vi "cal_cmd_to_string_position.vi"(0 "Last Function Ref In":refnum<vi>, 1 "Disable String":string="OFF", 2 "Enum":T1, 5 "Main Node BD Position":cluster{"Left":i32, "Top":i32}, 7 "1st sub node x position":i32, 9 "Last sub node y position/Offset":i32, 11 "error in (no error)":errorcluster) -> (4 "Last Function Ref Out":refnum<vi>, 6 "Main Node Position/Enable Constant Position":cluster{"Left":u32, "Top":i32}, 8 "Disable Constant Position":cluster{u32, i32}, 10 "1st sub node x position":i32, 15 "error out":errorcluster)   [LabVIEW 2018]
uses:
  TypeDefinitions/main_position_types.ctl
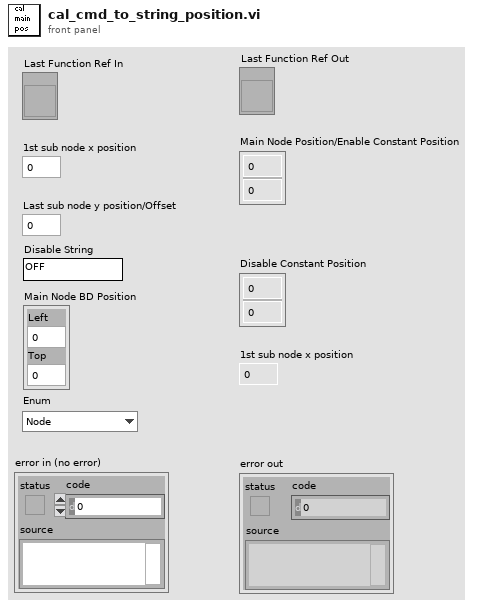
[diagram p1: front panel]
types:
  T1 = typedef "main_position_types.ctl" = enum16{"Node", "FormatNodeForMultipleControls", "BoolConstant", "FormatConstant", "1stSubNodeX"}
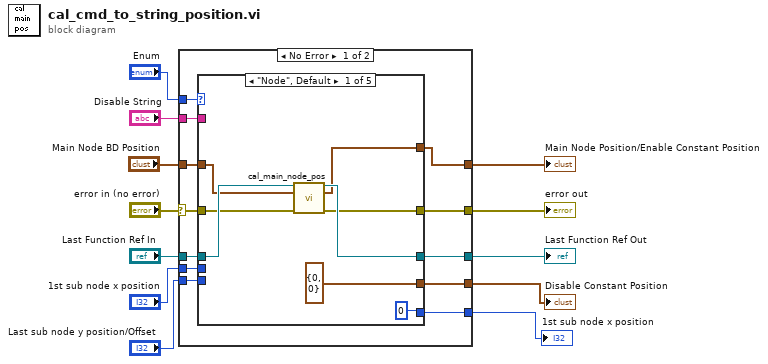
[diagram p0: block diagram]
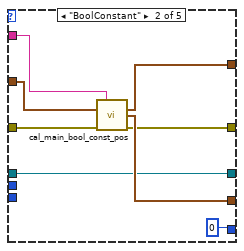
[diagram p2: hidden frame]
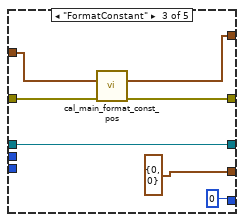
[diagram p3: hidden frame]
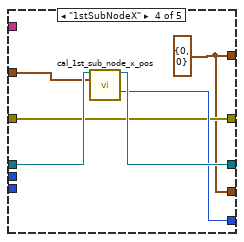
[diagram p4: hidden frame]
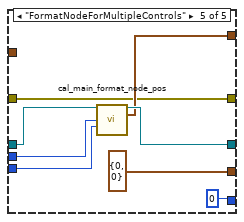
[diagram p5: hidden frame]
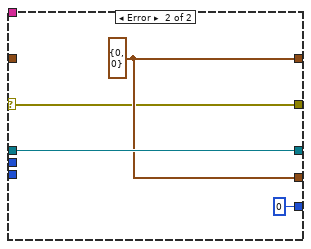
[diagram p6: hidden frame]
diagram:
  n1 = case shown="No Error" "error in (no error)" {
    selector: "error in (no error)" -> [w23 w63]
    tunnel: "Enum" -> [w24 _]
    tunnel: "Last Function Ref In" -> [w22 w65]
    tunnel: [w21 w65] -> w9
    tunnel: [w20 w64] -> w8
    tunnel: "1st sub node x position" -> [w19 _]
    tunnel: "Last sub node y position/Offset" -> [w18 _]
    tunnel: [w17 w63] -> w5
    tunnel: "Main Node BD Position" -> [w14 _]
    tunnel: "Disable String" -> [w16 _]
    tunnel: [w15 w64] -> w2
    tunnel: [w13 0 ("1st sub node x position")] -> w1
    frame No Error {
      n2 = case shown="\"Node\", Default" w24 {
        tunnel: w23 -> [w29 w36 w46 w49 w56]
        tunnel: w22 -> [w32 w34 w47 w53 w61]
        tunnel: [w31 w34 w47 w52 w60] -> w21
        tunnel: [w27 w38 w43 w48 w59] -> w20
        tunnel: w19 -> [_ _ _ _ w58]
        tunnel: w18 -> [_ _ _ _ w57]
        tunnel: [w28 w35 w45 w49 w56] -> w17
        tunnel: w14 -> [w30 w39 w44 w50 _]
        tunnel: w16 -> [_ w40 _ _ _]
        tunnel: [cluster{"Left":i32, "Top":i32} {"Left"=0, "Top"=0} ("Constant Position") w37 cluster{"Left":u32, "Top":i32} {"Left"=0, "Top"=0} ("Main Node Position") w48 cluster{"Left":i32, "Top":i32} {"Left"=0, "Top"=0} ("Constant Position")] -> w15
        tunnel: [0 ("1st sub node x position") 0 ("1st sub node x position") 0 ("1st sub node x position") w51 0 ("1st sub node x position")] -> w13
        frame "Node", Default {
          n3 = call "cal_main_node_pos.vi"("Last Function Ref"=w32, "Last Function Position"=w30, "error in (no error)"=w29) -> ("Last Function Ref Out"=w31:refnum<vi>, "BD Position"=w27:cluster{"Left":i32, "Top":i32}, "error out"=w28:errorcluster)  [unwired: 1 in, 9 out]
        }
        frame "BoolConstant" {
          n4 = call "cal_main_bool_const_pos.vi"("Disable String"=w40, "Main Node BD Position"=w39, "error in (no error)"=w36) -> ("Enable Constant Position"=w38:cluster{"Left":i32, "Top":i32}, "Disable Constant Position"=w37:cluster{"Left":i32, "Top":i32}, "error out"=w35:errorcluster)  [unwired: 10 out]
        }
        frame "FormatConstant" {
          n5 = call "cal_main_format_const_pos.vi"("Main Node BD Position"=w44, "error in (no error)"=w46) -> ("Constant Position"=w43:cluster{"Left":i32, "Top":i32}, "error out"=w45:errorcluster)  [unwired: 12 out]
        }
        frame "1stSubNodeX" {
          w48 = cluster{"Left":u32, "Top":i32} {"Left"=0, "Top"=0} ("Main Node Position")
          n6 = call "cal_1st_sub_node_x_pos.vi"("Last Function Ref In"=w53, "Last Function Position"=w50) -> ("Last Function Ref Out"=w52:refnum<vi>, "1st sub node x position"=w51:i32)  [unwired: 12 out]
        }
        frame "FormatNodeForMultipleControls" {
          n7 = call "cal_main_format_node_pos.vi"("Last Function Ref In"=w61, "1st sub node x position"=w58, "Last sub node y position"=w57) -> ("Last Function Ref Out"=w60:refnum<vi>, "Main Node Position"=w59:cluster{u32, i32})  [unwired: 11 out]
        }
      }
    }
    frame Error {
      w64 = cluster{"Left":i32, "Top":i32} {"Left"=0, "Top"=0} ("Constant Position")
    }
  }
  "Main Node Position/Enable Constant Position" <- w8
  "Last Function Ref Out" <- w9
  "error out" <- w5
  "Disable Constant Position" <- w2
  "1st sub node x position" <- w1
